vi "CreateNewMissions.vi"(4 "Timeout (s)":dbl, 6 "Duration (s)\n[For in-box mission]":dbl, 7 "Roundng Radius":dbl=15.0, 8 "Tolerance (m)":dbl, 9 "Mission Type":T3, 10 "Points of Interest":T4[](array[typedef]) {"North" format="%#_10f"; "East" format="%#_8f"}, 11 "Initialized Mission Arrays":T1 {"Readable Missions"."Points of Interest"."North" format="%#_10f"; "Readable Missions"."Points of Interest"."East" format="%#_8f"}) -> (2 "New Mission OUT":refnum<class "GenericMission.lvclass">, 3 "Mission Array Cluster":T1 {"Readable Missions"."Points of Interest"."North" format="%#_10f"; "Readable Missions"."Points of Interest"."East" format="%#_8f"})   [LabVIEW 2013]
doc: "This VI takes in the indicated Mission type and necessary parameters, then creates the Mission object and adds it to\n1) The human readable mission array and\n2) The actual array of mission objects\n\nEric Schneider, August 2014"
uses:
  cRIO_Code/Data/TypeDefs/UTM Location.ctl
  cRIO_Code/Logic/Classes/Missions/GenericMission/GenericMission.lvclass
  cRIO_Code/Data/TypeDefs/MissionTypeControl.ctl
  TypeDef/mission_arrays.ctl
  cRIO_Code/Data/TypeDefs/MissionDescription.ctl
  cRIO_Code/Logic/Classes/Missions/GoTo/GoTo.lvclass
  cRIO_Code/Logic/Classes/Missions/RoundBouy/RoundBouy.lvclass
  cRIO_Code/Logic/Classes/Missions/PassBouy/PassBouy.lvclass
  cRIO_Code/Logic/Classes/Missions/StationKeeping/StationKeeping.lvclass
  cRIO_Code/Logic/Classes/Missions/RoundBouy/RoundBouy.lvclass/RoundBouy.ctl
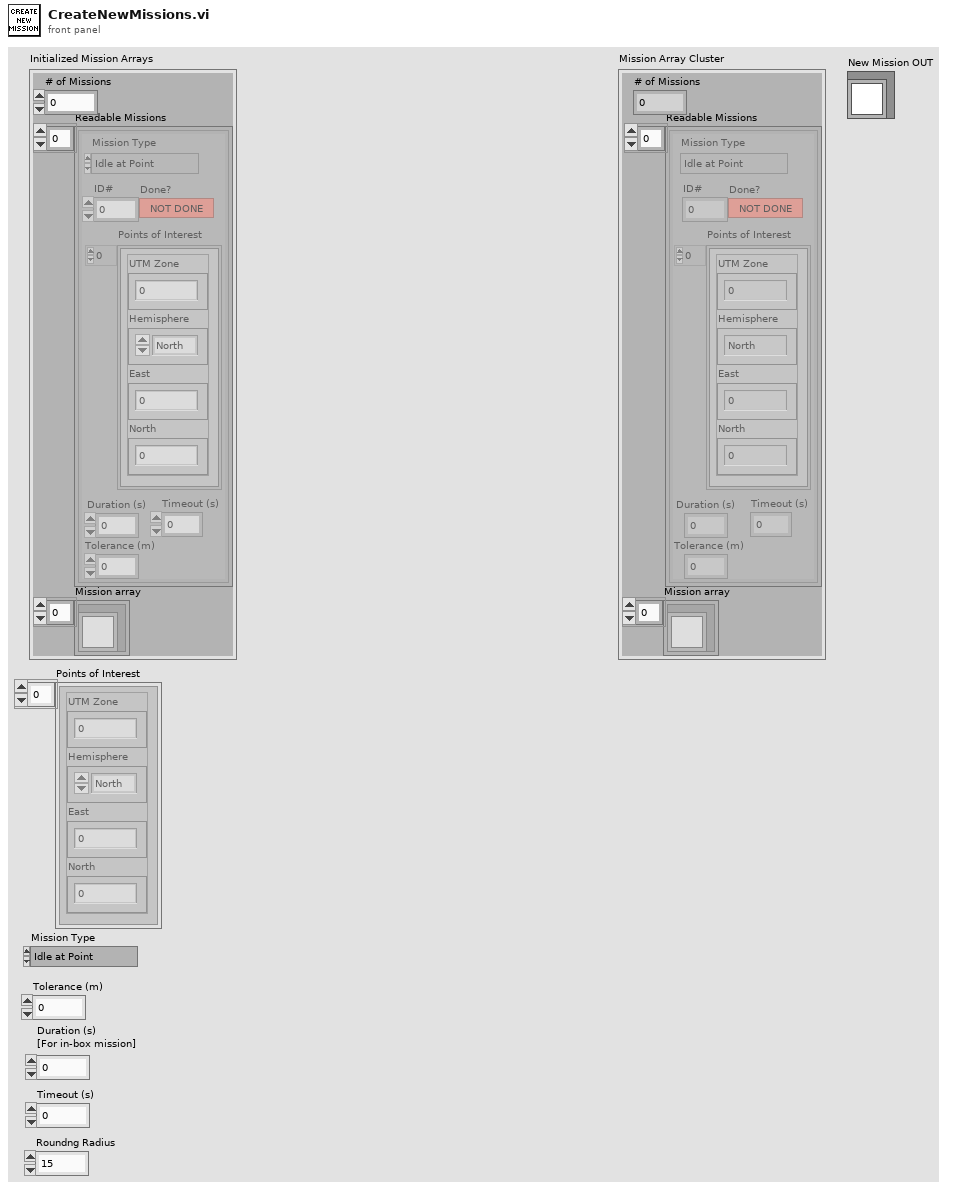
[diagram p1: front panel]
types:
  T1 = typedef "mission_arrays.ctl" = cluster{"# of Missions":i32, "Readable Missions":T2[], "Mission array":refnum<class "GenericMission.lvclass">[]}
  T2 = typedef "MissionDescription.ctl" = cluster{"Duration (s)":dbl, "Timeout (s)":dbl, "Tolerance (m)":dbl, "Mission Type":T3, "Points of Interest":T4[], "ID#":i32, "Done?":bool}
  T3 = typedef "MissionTypeControl.ctl" = enum16{"Idle at Point", "Drive to Waypoint", "Round Buoy to Port", "Round Buoy to Starboard", "Pass Between Buoys", "Station Keeping"}
  T4 = typedef "UTM Location.ctl" = cluster{"UTM Zone":dbl, "Hemisphere":enum16{"North", "South"}, "East":dbl, "North":dbl}
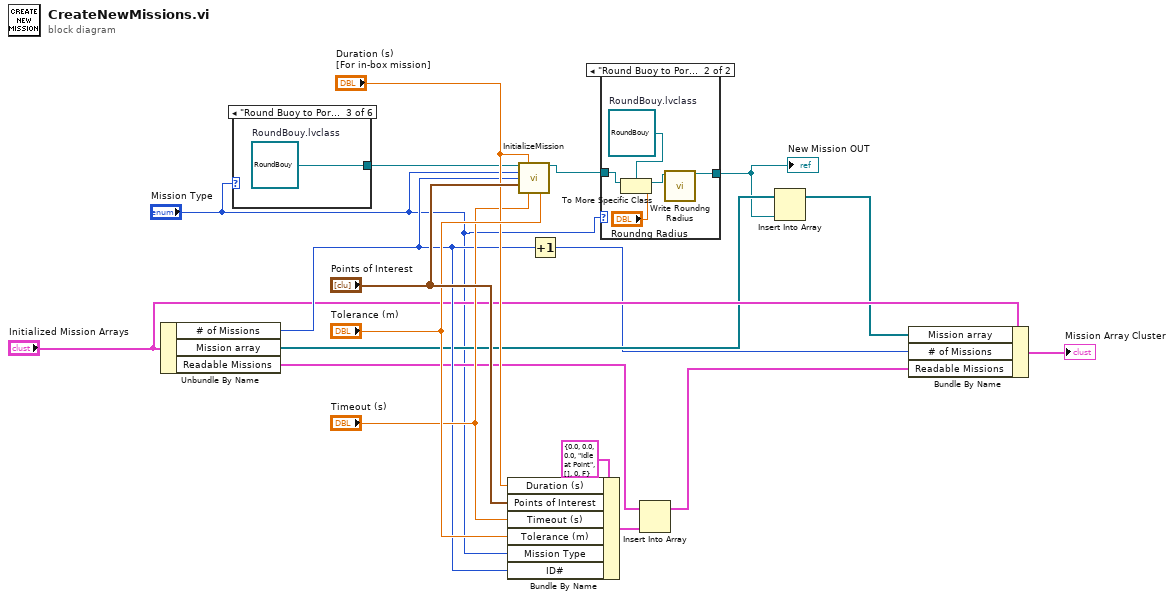
[diagram p0: block diagram]
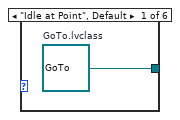
[diagram p3: hidden frame]
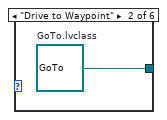
[diagram p4: hidden frame]
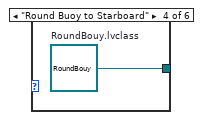
[diagram p5: hidden frame]
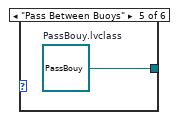
[diagram p6: hidden frame]
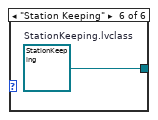
[diagram p7: hidden frame]
diagram:
  n1 = Unbundle By Name("Initialized Mission Arrays") -> ("# of Missions"=w11:i32, "Mission array"=w9:refnum<class "GenericMission.lvclass">[], "Readable Missions"=w8:T2[])
  n2 = case shown="\"Round Buoy to Port\"" "Mission Type" {
    tunnel: [w19 w20 w21 w22 w23 w24] -> w12
    frame "Idle at Point", Default {
      w19 = refnum<class "GoTo.lvclass"> refnum  # GoTo.lvclass
    }
    frame "Drive to Waypoint" {
      w20 = refnum<class "GoTo.lvclass"> refnum  # GoTo.lvclass
    }
    frame "Round Buoy to Port" {
      w21 = refnum<class "RoundBouy.lvclass"> refnum  # RoundBouy.lvclass
    }
    frame "Round Buoy to Starboard" {
      w22 = refnum<class "RoundBouy.lvclass"> refnum  # RoundBouy.lvclass
    }
    frame "Pass Between Buoys" {
      w23 = refnum<class "PassBouy.lvclass"> refnum  # PassBouy.lvclass
    }
    frame "Station Keeping" {
      w24 = refnum<class "StationKeeping.lvclass"> refnum  # StationKeeping.lvclass
    }
  }
  n3 = Bundle By Name(cluster=T2 {"Duration (s)"=0.0, "Timeout (s)"=0.0, "Tolerance (m)"=0.0, "Mission Type"=enum."Idle at Point", "Points of Interest"=[], "ID#"=0, "Done?"=FALSE} ("input cluster"), "Duration (s)"="Duration (s)\n[For in-box mission]", "Points of Interest"="Points of Interest", "Timeout (s)"="Timeout (s)", "Tolerance (m)"="Tolerance (m)", "Mission Type"="Mission Type", "ID#"=w11) -> (w14:T2)
  n4 = call-dynamic "InitializeMission.vi"("GenericMission in"=w12, "Duration (s)"="Duration (s)\n[For in-box mission]", "Mission Type"="Mission Type", "ID#"=w11, "Points of Interest"="Points of Interest", "Timeout (s)"="Timeout (s)", "Tolerance (m)"="Tolerance (m)") -> ("GenericMission out"=w2:refnum<class "GenericMission.lvclass">)  [unwired: 7 in, 1 out]
  n5 = Increment(x=w11) -> (x+1=w6:i32)
  n6 = case shown="\"Round Buoy to Port\", \"Round Buoy to Starboard\"" "Mission Type" {
    tunnel: w2 -> [w25 w29]
    tunnel: [w25 w30] -> w1
    frame "Idle at Point", Default {
    }
    frame "Round Buoy to Port", "Round Buoy to Starboard" {
      w28 = refnum<class "RoundBouy.lvclass"> refnum  # RoundBouy.lvclass
      n7 = To More Specific Class(target class=w28, reference=w29) -> (specific class reference=w27:refnum<class "RoundBouy.lvclass">)  [unwired: 1 in, 1 out]
      n8 = call "Write Roundng Radius.vi"("Roundng Radius"="Roundng Radius", "RoundBouy in"=w27) -> ("RoundBouy out"=w30:refnum<class "RoundBouy.lvclass">)  [unwired: 8 in, 1 out]
    }
  }
  "New Mission OUT" <- w1
  n9 = Insert Into Array(array=w8, new element=w14) -> (w7:T2[])  [unwired: 1 in]
  n10 = Insert Into Array(array=w9, new element=w1) -> (w5:refnum<class "GenericMission.lvclass">[])  [unwired: 1 in]
  n11 = Bundle By Name(cluster="Initialized Mission Arrays", "Mission array"=w5, "# of Missions"=w6, "Readable Missions"=w7) -> (→"Mission Array Cluster":T1)
